vi "Get Stream.vi"(8 "error in (no error)":errorcluster, 11 "Connection in":refnum<class "Connection.lvclass">) -> (0 "error out":errorcluster, 2 "Stream":refnum<class "Stream.lvclass">, 3 "Connection out":refnum<class "Connection.lvclass">)   [LabVIEW 2020, in "Stream.lvlib" / "Connection.lvclass"]
doc: "Returns the stream implementation that can be used to read & write data to this connection."
uses:
  Connection.lvclass
  Stream.lvlib
  Stream/Stream.lvclass
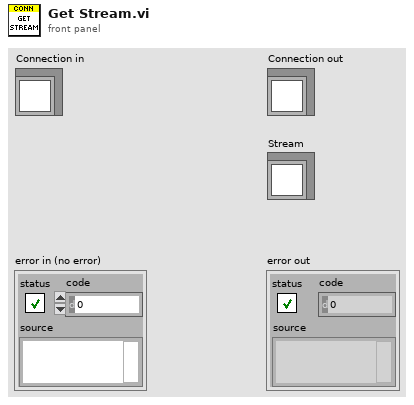
[diagram p1: front panel]
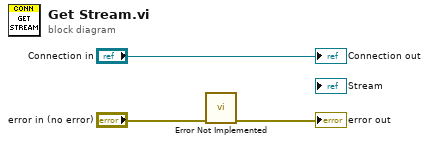
[diagram p0: block diagram]
diagram:
  n1 = call "Error Not Implemented.vi"("error in (no error)"="error in (no error)") -> ("error out"=→"error out":errorcluster)  [unwired: 10 in]
  "Connection out" <- "Connection in"
